vi "Make shift data.vi"(0 "startphases":i32=3, 1 "reps":i32=2 caption="Repetitions", 3 "randomize":bool=TRUE, 5 "endphases":i32=3, 7 "sinfreq":dbl=1.5 caption="sinefreq", 11 "Durations":dbl[](array[numeric])=[0.2], 12 "pre cycles":dbl=10.0 caption="Pre cycles", 13 "post cycles":dbl=10.0 caption="Post cycles", 14 "cyclesperpulse":dbl=10.0 caption="Cycles per pulse") -> (4 "pulse data":T1, 6 "totaltime":dbl caption="Total time")   [LabVIEW 2013]
uses:
  Pulse data.ctl
  <vilib>/gmath/statdist.llb/Random Permutation.vi
  <vilib>/gmath/NI_Gmath.lvlib
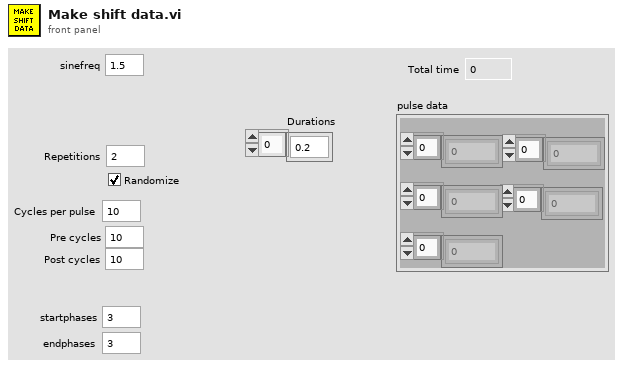
[diagram p1: front panel]
types:
  T1 = typedef "Pulse data.ctl" = cluster{"time":dbl[], "phase":dbl[], "dir/shift":dbl[], "amplitude":dbl[], "duration":dbl[]}
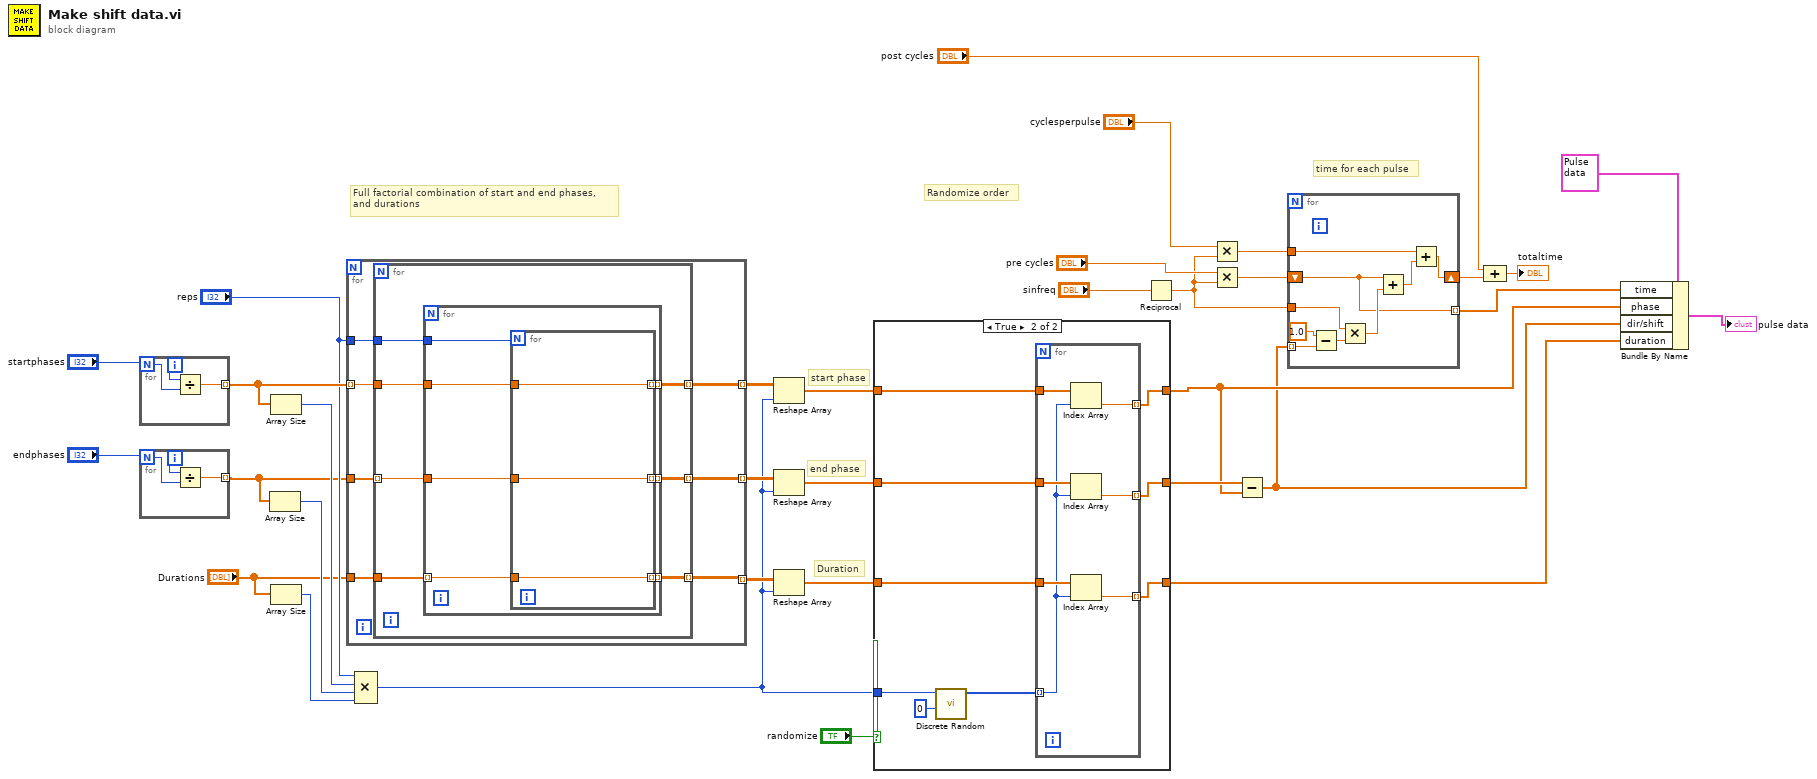
[diagram p0: block diagram]
diagram:
  # "end phase"
  # "time for each pulse"
  # "Duration"
  # "start phase"
  # "Randomize order"
  # "Full factorial combination of start and end phases,\nand durations"
  n1 = for {
    N: "startphases" -> [w36]
    tunnel: [w34] -> w31 mode=indexing
    i -> [w35]
    n2 = Divide(x=w35, y=w36) -> (x/y=w34:dbl)
  }
  n3 = for {
    N: "endphases" -> [w39]
    tunnel: [w37] -> w5 mode=indexing
    i -> [w38]
    n4 = Divide(x=w38, y=w39) -> (x/y=w37:dbl)
  }
  n5 = Array Size(array=w5) -> (size(s)=w30:i32)
  n6 = Array Size(array=w31) -> (size(s)=w29:i32)
  n7 = Array Size(array="Durations") -> (size(s)=w22:i32)
  n8 = for {
    tunnel: w31 -> [w44] mode=indexing
    tunnel: w5 -> [w46]
    tunnel: "reps" -> [w45]
    tunnel: [w43] -> w32 mode=indexing
    tunnel: [w42] -> w27 mode=indexing
    tunnel: [w41] -> w21 mode=indexing
    tunnel: "Durations" -> [w40]
    n9 = for {
      tunnel: w46 -> [w51] mode=indexing
      tunnel: w45 -> [w53]
      tunnel: w44 -> [w52]
      tunnel: [w50] -> w43 mode=indexing
      tunnel: [w49] -> w42 mode=indexing
      tunnel: [w48] -> w41 mode=indexing
      tunnel: w40 -> [w47]
      n10 = for {
        tunnel: w53 -> [w60]
        tunnel: w52 -> [w59]
        tunnel: w51 -> [w58]
        tunnel: [w57] -> w50 mode=indexing
        tunnel: [w56] -> w49 mode=indexing
        tunnel: [w55] -> w48 mode=indexing
        tunnel: w47 -> [w54] mode=indexing
        n11 = for {
          N: w60 -> [_]
          tunnel: w59 -> [w63]
          tunnel: w58 -> [w62]
          tunnel: [w63] -> w57 mode=indexing
          tunnel: [w62] -> w56 mode=indexing
          tunnel: [w61] -> w55 mode=indexing
          tunnel: w54 -> [w61]
        }
      }
    }
  }
  n12 = Compound Arithmetic op=MULTIPLY("reps", w29, w30, w22) -> (w20:i32)
  n13 = Reshape Array(w32, w20) -> (w25:dbl[])
  n14 = Reshape Array(w27, w20) -> (w24:dbl[])
  n15 = Reshape Array(w21, w20) -> (w19:dbl[])
  n16 = case shown="True" "randomize" {
    tunnel: w20 -> [_ w74]
    tunnel: w25 -> [w66 w73]
    tunnel: w24 -> [w65 w72]
    tunnel: [w66 w69] -> w2
    tunnel: [w65 w70] -> w3
    tunnel: w19 -> [w64 w68]
    tunnel: [w64 w67] -> w17
    frame False {
    }
    frame True {
      n17 = call-poly <vilib>:"Discrete Random.vi"("start"=0, "N"=w74) -> ("random permutation"=w71:i32[])  [unwired: 8 in, 1 out]
      n18 = for {
        tunnel: w73 -> [w82]
        tunnel: w72 -> [w81]
        tunnel: w71 -> [w76] mode=indexing
        tunnel: [w80] -> w69 mode=indexing
        tunnel: [w79] -> w70 mode=indexing
        tunnel: w68 -> [w78]
        tunnel: [w77] -> w67 mode=indexing
        n19 = Index Array(array=w82, index=w76) -> (element=w80:dbl)
        n20 = Index Array(array=w81, index=w76) -> (element=w79:dbl)
        n21 = Index Array(array=w78, index=w76) -> (element=w77:dbl)
      }
    }
  }
  n22 = Reciprocal(x="sinfreq") -> (1/x=w4:dbl)
  n23 = Multiply(x="cyclesperpulse", y=w4) -> (x*y=w10:dbl)
  n24 = Multiply(x="pre cycles", y=w4) -> (x*y=w8:dbl)
  n25 = Subtract(x=w3, y=w2) -> (x-y=w1:dbl[])
  n26 = for {
    tunnel: w10 -> [w91]
    tunnel: [w83] -> w18 mode=indexing
    shift-right: [w90] -> w7
    shift-left: w8 -> [w83]
    tunnel: w1 -> [w89] mode=indexing
    tunnel: w4 -> [w86]
    n27 = Subtract(x=1.0, y=w89) -> (x-y=w87:dbl)
    n28 = Multiply(x=w86, y=w87) -> (x*y=w85:dbl)
    n29 = Add(x=w83, y=w85) -> (x+y=w84:dbl)
    n30 = Add(x=w91, y=w84) -> (x+y=w90:dbl)
  }
  n31 = Compound Arithmetic op=ADD("post cycles", w7) -> (→"totaltime":dbl)
  n32 = Bundle By Name(cluster=T1 {"time"=[0.2222222222222222, 6.888888888888888, 13.333333333333332, 20.22222222222222, 26.666666666666664, 33.77777777777777, 40.44444444444444, 46.666666666666664, 53.77777777777777, 59.99999999999999, 66.88888888888889, 73.77777777777777], "phase"=[0.3333333333333333, 0.3333333333333333, 0.0, 0.3333333333333333, 0.0, 0.6666666666666666, 0.6666666666666666, 0.0, 0.6666666666666666, 0.0, 0.3333333333333333, 0.6666666666666666], "dir/shift"=[1.0, -1.0, -1.0, 1.0, 1.0, -1.0, -1.0, -1.0, 1.0, 1.0, -1.0, 1.0], "amplitude"=[5.0, 5.0, 5.0, 5.0, 5.0, 5.0, 5.0, 5.0, 5.0, 5.0, 5.0, 5.0], "duration"=[0.2, 0.2, 0.2, 0.2, 0.2, 0.2, 0.2, 0.2, 0.2, 0.2, 0.2, 0.2]} ("pulse data 2"), "time"=w18, "phase"=w2, "dir/shift"=w1, "duration"=w17) -> (→"pulse data":T1)
